vi "Meas PowerSupply.vi"(0 "address string":string="8", 2 "error in (no error)":errorcluster) -> (3 "address string 2":string="8", 4 "Voltage":dbl[unit], 5 "Current":dbl[unit], 6 "error out":errorcluster)   [LabVIEW 2017]
panel:
  in  "Enable":bool=TRUE
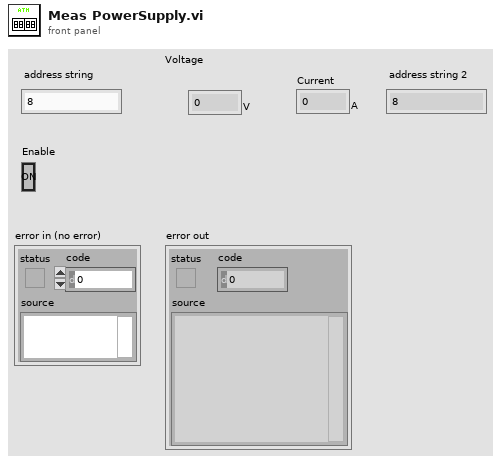
[diagram p1: front panel]
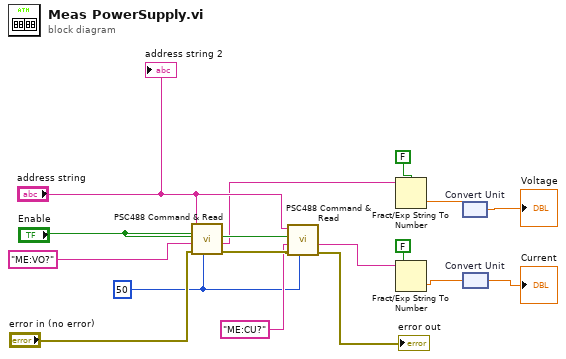
[diagram p0: block diagram]
diagram:
  w1 = u16 50 ("write/Read delay")
  n1 = call "PSC488 Command & Read.vi"("write/Read delay"=w1, "error in (no error)"="error in (no error)", "Com.string"="ME:VO?", "Enable"="Enable", "ADDRESS"="address string") -> ("error out"=w12:errorcluster, "String Out"=w5:string)  [unwired: 1 in, 3 out]
  n2 = call "PSC488 Command & Read.vi"("write/Read delay"=w1, "error in (no error)"=w12, "Com.string"="ME:CU?", "Enable"="Enable", "ADDRESS"="address string") -> ("error out"=→"error out":errorcluster, "String Out"=w9:string)  [unwired: 1 in, 3 out]
  n3 = Fract/Exp String To Number(use system decimal point (T)=FALSE, string=w5) -> (number=w3:dbl)  [unwired: 2 in, 1 out]
  n4 = Fract/Exp String To Number(use system decimal point (T)=FALSE, string=w9) -> (number=w7:dbl)  [unwired: 2 in, 1 out]
  n5 = node "Convert Unit"(w3) -> (→"Voltage":dbl[unit])
  n6 = node "Convert Unit"(w7) -> (→"Current":dbl[unit])
  "address string 2" <- "address string"
